vi "Ballard 429 - Clean-up.vi"(0 "Card Parameters (in)":T1, 11 "Error (in)":errorcluster) -> (15 "Error (out)":errorcluster)   [LabVIEW 2017, in "Ballard Arinc-429 Engine.lvlib"]
uses:
  Ballard Arinc-429 Engine.lvlib
  RT Controls/Card Parameters.ctl
  <instrlib>/BTICardLib/BTICardLV.lvlib
  <instrlib>/BTI429Lib/BTI429LV.lvlib
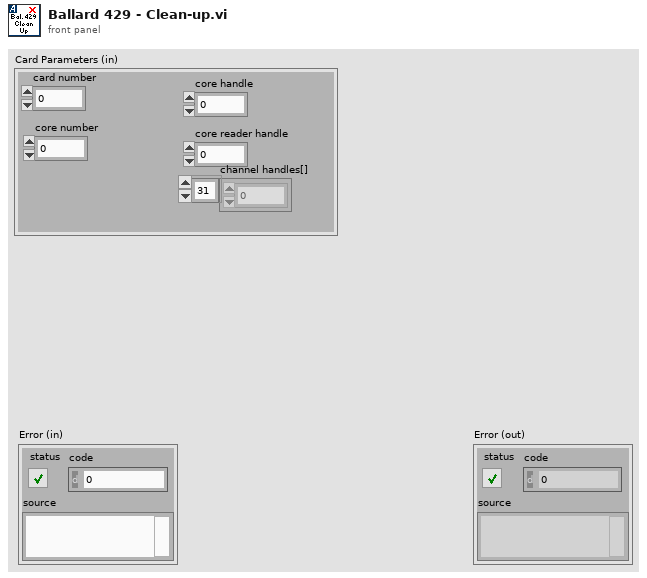
[diagram p1: front panel]
types:
  T1 = typedef "Ballard Arinc-429 Engine.lvlib/Card Parameters.ctl" = cluster{"card number":i32, "core number":i32, "core handle":u64, "core reader handle":u64, "channel handles[]":u64[]}
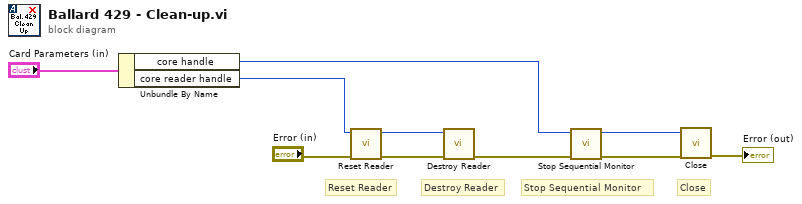
[diagram p0: block diagram]
diagram:
  # "Destroy Reader"
  # "Close"
  # "Stop Sequential Monitor"
  # "Reset Reader"
  n1 = Unbundle By Name("Card Parameters (in)") -> ("core handle"=w6:u64, "core reader handle"=w7:u64)
  n2 = call <instrlib>:"Reset Reader.vi"("error in (no error)"="Error (in)", "reader handle in"=w7) -> ("error out"=w3:errorcluster, "reader handle out"=w1:u64)  [unwired: 8 in]
  n3 = call <instrlib>:"Destroy Reader.vi"("error in (no error)"=w3, "reader handle in"=w1) -> ("error out"=w2:errorcluster)  [unwired: 9 in]
  n4 = call <instrlib>:"Stop Sequential Monitor.vi"("error in (no error)"=w2, "core handle in"=w6) -> ("error out"=w9:errorcluster, "core handle out"=w10:u64)  [unwired: 8 in]
  n5 = call <instrlib>:"Close.vi"("error in (no error)"=w9, "core handle in"=w10) -> ("error out"=→"Error (out)":errorcluster)  [unwired: 8 in, 1 out]
